vi "DAC_set_value.vi"(1 "InstInfo":T2, 2 "FPGA Ref":T1, 3 "Point":T3) -> (0 "FPGA VI Reference Out":T1)   [LabVIEW 2013]
uses:
  fpga-bitfile-ref.ctl
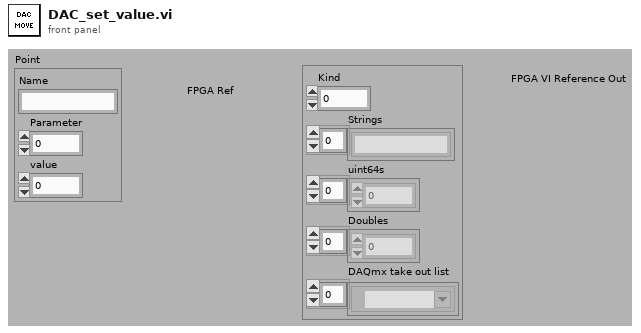
[diagram p1: front panel]
types:
  T1 = typedef "fpga-bitfile-ref.ctl" = refnum<k20>
  T2 = cluster{"Kind":u16, "Strings":string[], "uint64s":u64[], "Doubles":dbl[], "DAQmx take out list":refnum<k21>[]}
  T3 = cluster{"Name":string, "Parameter":u16, "value":dbl}
  T4 = enum8{"start movement", "buses to use", "delay", "value"}
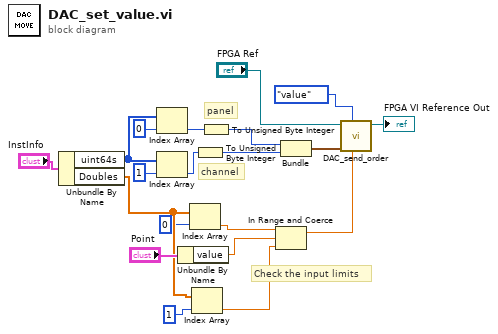
[diagram p0: block diagram]
diagram:
  # "Check the input limits"
  # "channel"
  # "panel"
  n1 = Unbundle By Name("InstInfo") -> ("uint64s"=w18:u64[], "Doubles"=w5:dbl[])
  n2 = Index Array(array=w18, index=0) -> (element=w15:u64)
  n3 = Index Array(array=w18, index=1) -> (element=w14:u64)
  n4 = Unbundle By Name("Point") -> ("value"=w7:dbl)
  n5 = Index Array(array=w5, index=0) -> (element=w1:dbl)
  n6 = Index Array(array=w5, index=1) -> (element=w2:dbl)
  n7 = To Unsigned Byte Integer(number=w14) -> (unsigned 8bit integer=w12:u8)
  n8 = To Unsigned Byte Integer(number=w15) -> (unsigned 8bit integer=w13:u8)
  n9 = In Range and Coerce(upper limit=w1, x=w7, lower limit=w2) -> (coerced(x)=w6:dbl)  [unwired: 1 out]
  n10 = Bundle(w13, w12) -> (w10:cluster{u8, u8})  [unwired: 1 in]
  n11 = call "DAC_send_order.vi"("DAC goto value"=w6, "order"=T4."value", "Cluster"=w10, "FPGA VI Reference In"="FPGA Ref") -> ("FPGA VI Reference Out"=→"FPGA VI Reference Out":T1)  [unwired: 3 in, 4 out]
